vi "Main_Equip_Refo_ref749.vi"() -> ()   [LabVIEW 2017]
panel:
  out "TempeSenseTara":sgl caption="Temperature" format="%.1f"
  out "Temps SenseTara":sgl caption="Time" format="%.1f"
  out "TaraTemp":sgl[](array[numeric])
  in  "Test Selection":enum32{"Delta T", "EPI Calibration"}(radio)
  out "Pendent":sgl caption="Gradient :" format="%.2f"
  out "hardware name":string
  out "isOnline 2":bool
  out "IndexSup":i32
  out "IndexInf":i32
  in  "Verifica":bool
  out "High Time":sgl format="%#_3g"
  out "Low Time":sgl format="%#_3g"
  in  "High Temp.":sgl
  in  "Low Temp.":sgl
  out "Temps":sgl caption="Time" format="%.1f"
  out "Calibration result:":bool
  out "error out_USB":errorcluster
  out "Nom Sensor Temperatura":string
  in  "Dades":sgl[](array[numeric])
  in  "Guardar 24h":bool caption="Informe"
  out "Dies":u8 caption="NumDies"
  in  "Reset_AutoSave 24":bool
  in  "mT1":sgl caption="Temperatura_1" format="%.1f"
  out "Maxim":sgl
  in  "BtSalir":bool caption="Sortir"
  in  "Reset_AutoSave":bool
  in  "Test name:":string
  out "Gràfiques T-Temps":cluster{"Value":sgl[], "Value":sgl[]}[](graph)
  in  "Datos OK":bool
  out "DadesComplertes":sgl[](array[numeric])
  in  "Grafica_OK":bool=TRUE
  out "Tabla":sgl[][](array[numeric])
  in  "Registro OK":bool=TRUE
  in  "time out":bool
  in  "Reset_gráfica":bool
  in  "Reset_Time":bool
  in  "Tiempo_string":string[](array[string])
  out "Elapsed Time (s)":i32
  out "Ensayo activo":bool
  out "FSenseTara":sgl caption="Fuerza - N"
  in  "CaptadorF":u16(ring) caption="Unidades" items=["25kg"=5]
  in  "PendentLlum":sgl caption="Força" format="%.1f"
  out "FactorsUnitatsPendents_F":dbl[](array[numeric])
  out "ConversioUnitatsF":dbl[](array[numeric])=[1.0, 9.8756, 2.2]
  out "ArraiUnitats":cluster{"String":string, "Value":u16}[](array[cluster])=[{"String"="kg", "Value"=0}, {"String"="N", "Value"=1}, {"String"="g", "Value"=2}, {"String"="daN", "Value"=3}, {"String"="cN", "Value"=4}, {"String"="KN", "Value"=5}, {"String"="lb", "Value"=6}]
  out "Tara":sgl caption="Força" format="%.1f"
  out "Temperatura1":sgl caption="Temperature" format="%.1f"
  out "PendentsT":sgl[](array[numeric])
  in  "Salir":bool caption="Sortir"
  in  "Ensayonuevo":bool caption="New Test"
  in  "Guardar":bool
  in  "Iniciar / Finalizar":bool=TRUE caption="Finalitzar prova"
  in  "UnidadesF":u16(ring) caption="Unidades" items=["kg", "N", "g"]
  out "FirstTime?":bool caption="TARA"
  # "s"
  # "ºC / s"
  # "ºC"
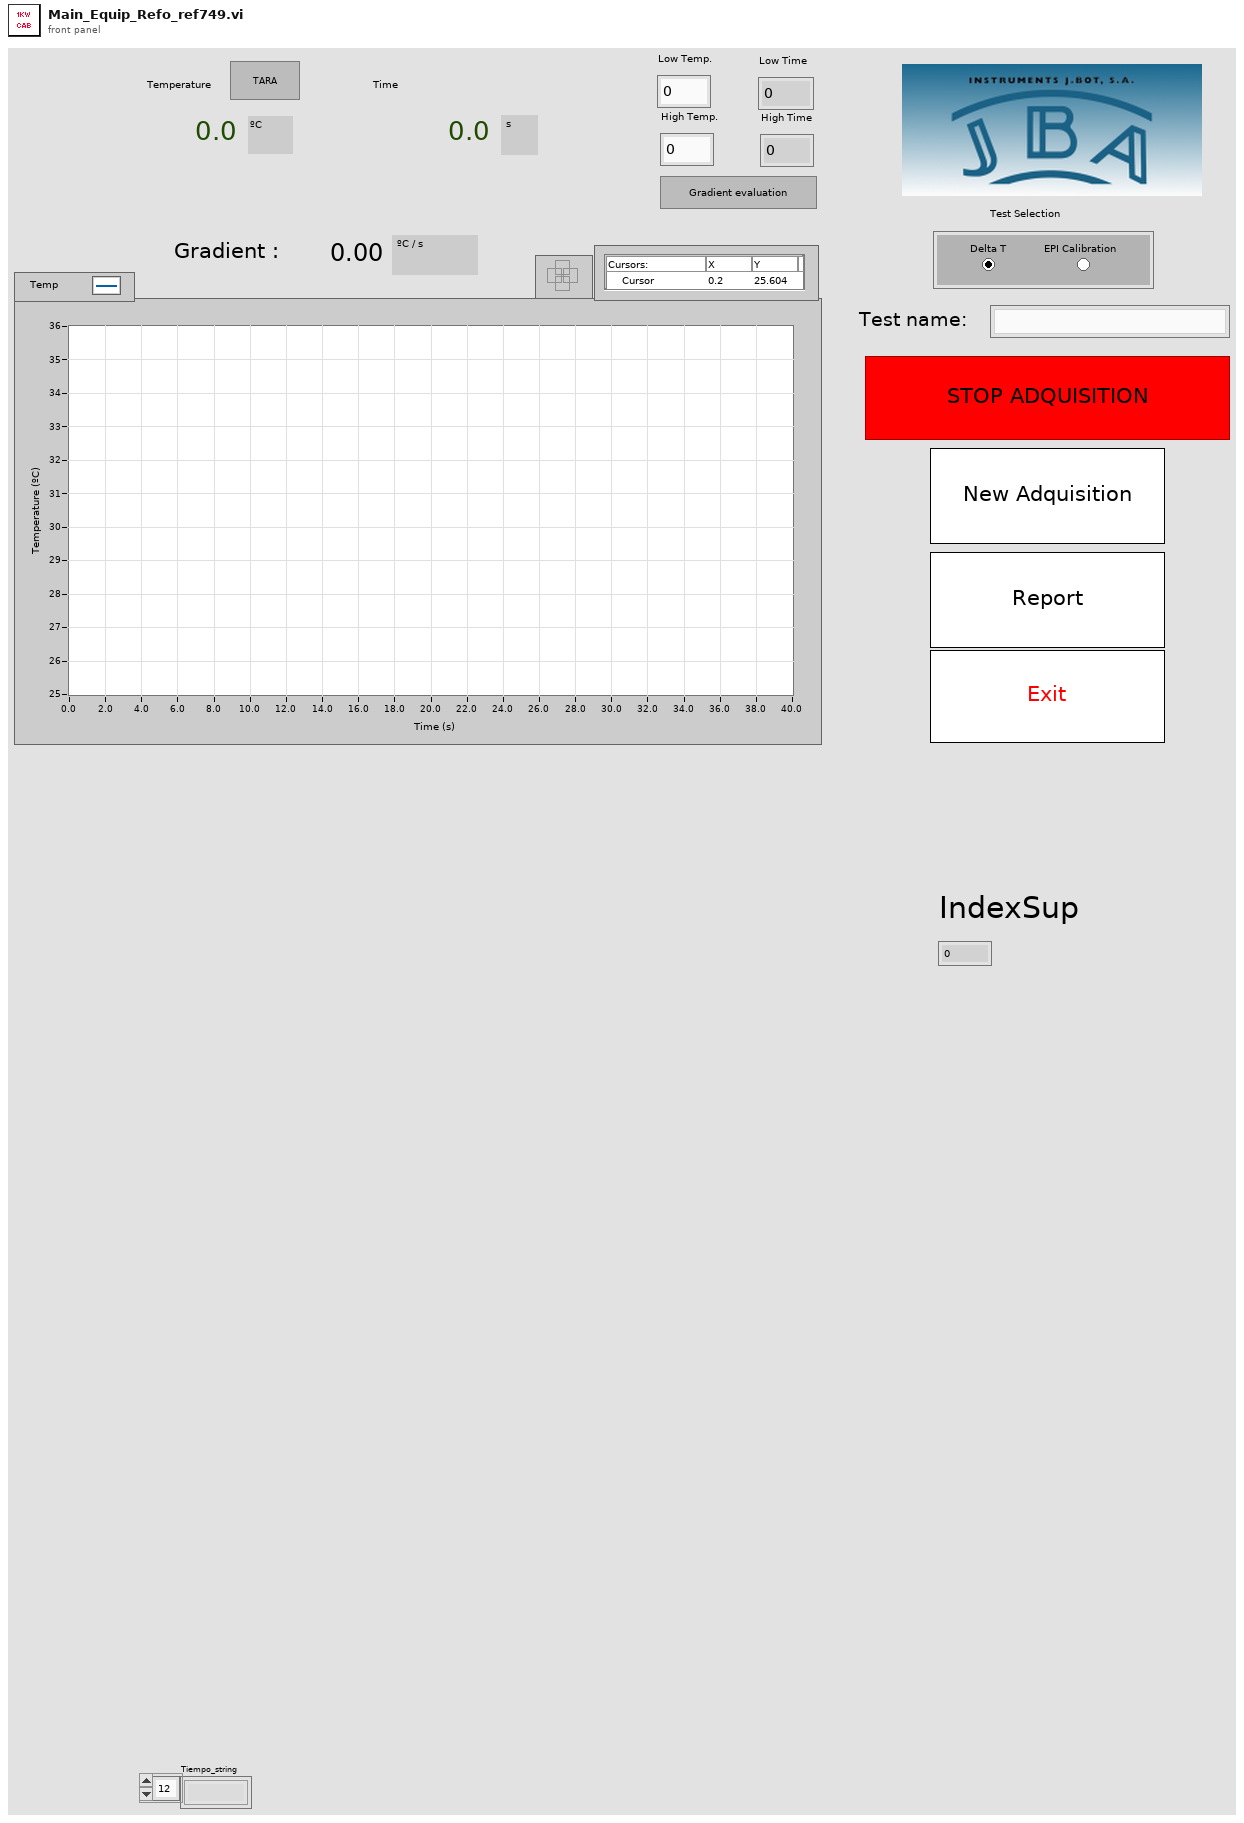
[diagram p1: front panel]
types:
  T1 = enum8{"Enabled", "Disabled", "Disabled and Grayed Out"}
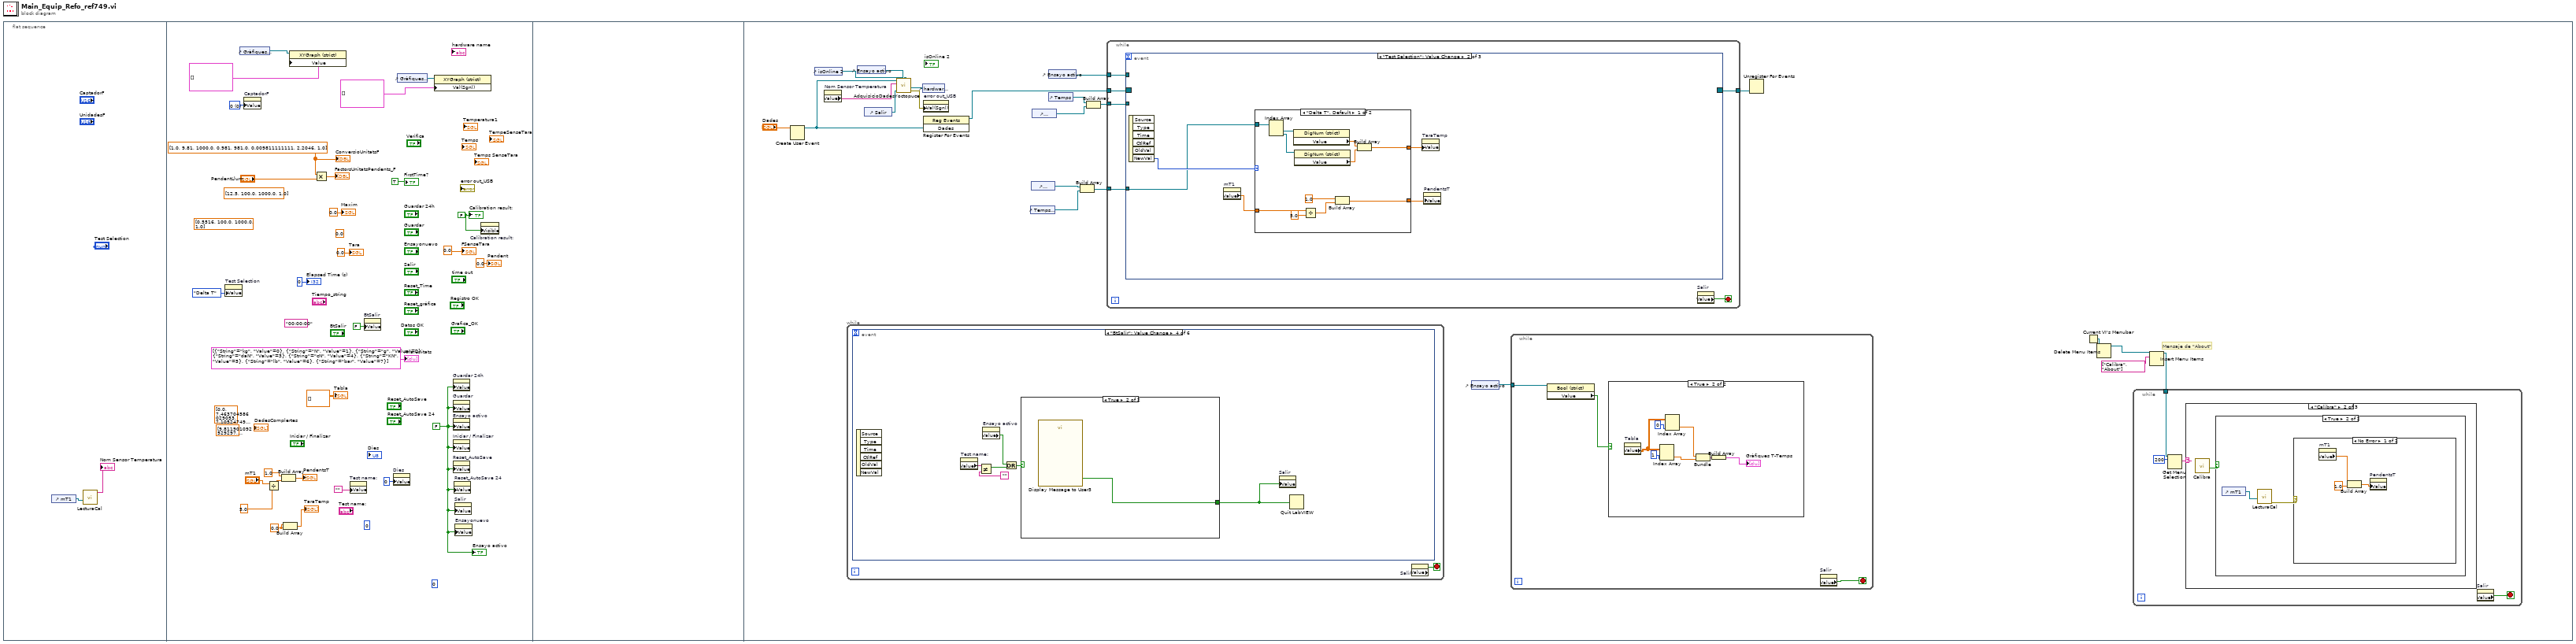
[diagram p0: block diagram]
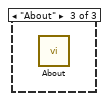
[diagram p5: hidden frame]
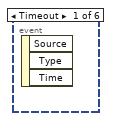
[diagram p7: hidden frame]
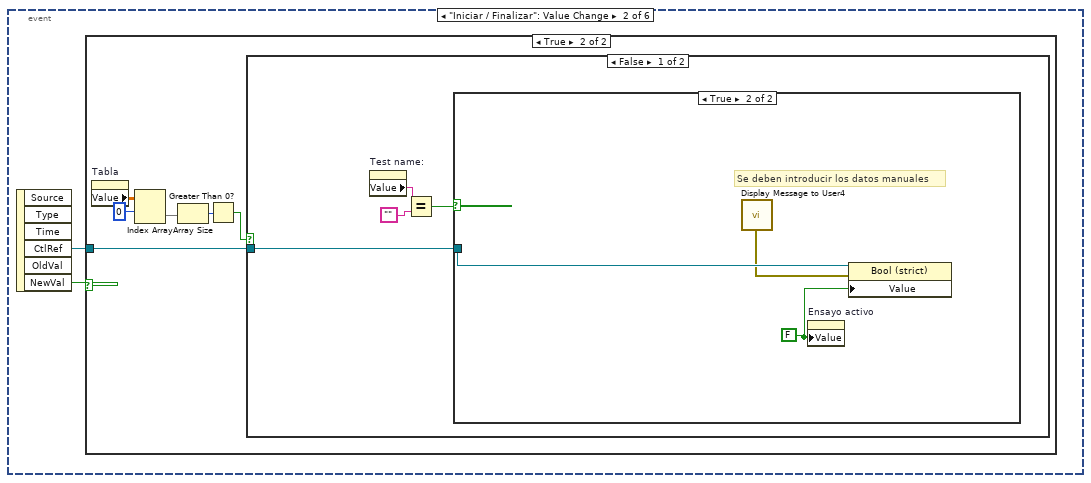
[diagram p8: hidden frame]
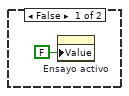
[diagram p9: hidden frame]
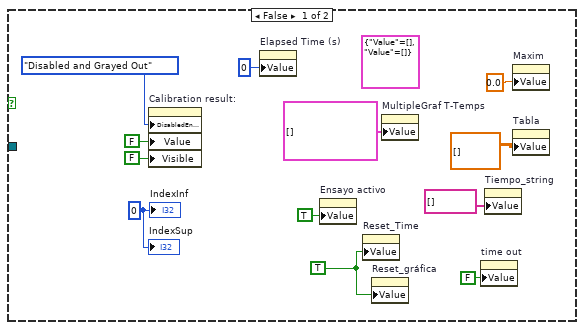
[diagram p10: hidden frame]
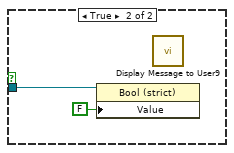
[diagram p11: hidden frame]
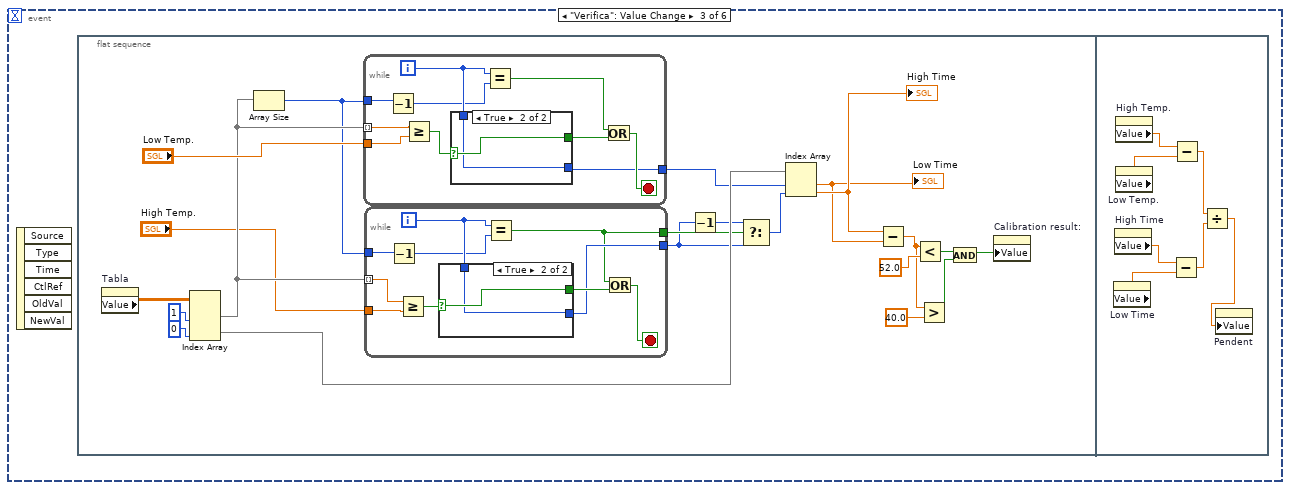
[diagram p12: hidden frame]
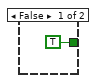
[diagram p15: hidden frame]
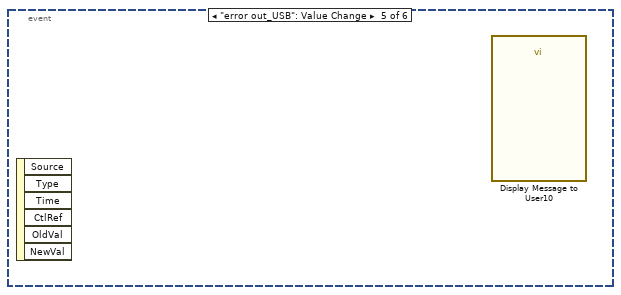
[diagram p16: hidden frame]
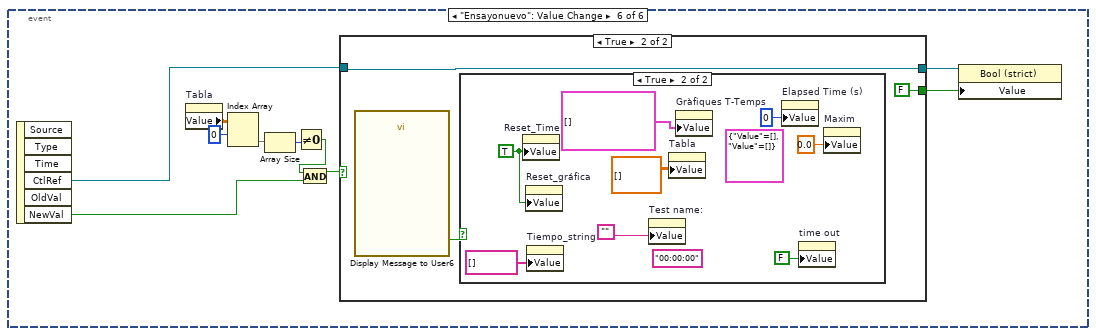
[diagram p17: hidden frame]
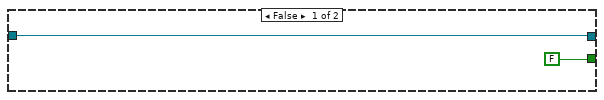
[diagram p18: hidden frame]
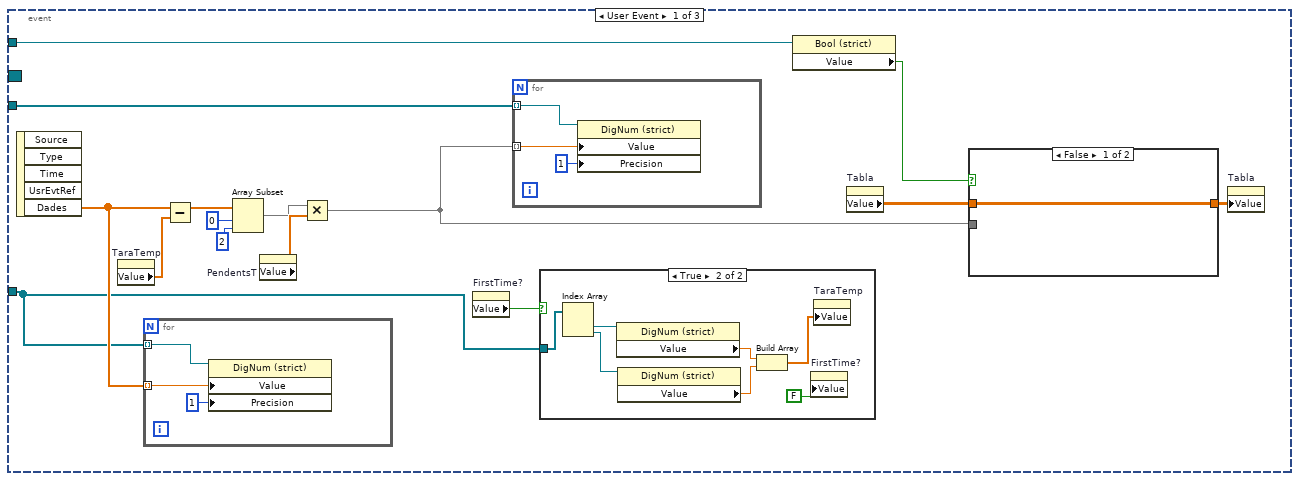
[diagram p20: hidden frame]
diagram:
  n1 = flat-sequence {
    frame #0 {
      n2 = control-ref of="mT1"() -> (w2:refnum<vi>)
      n3 = call "LecturaCal.vi"("T1"=w2) -> ("Nom Sensor Temperatura"=→"Nom Sensor Temperatura":string)  [unwired: 9 in, 1 out]
    }
    frame #1 {
      w10 = 0.0 ("element")
      w12 = FALSE ("Resultat Assaig")
      (unwired) sgl[] [9.811901, 9.763803, 9.671529, 9.535354] ("DadesComplertes")
      (unwired) sgl[][] [[0.0, 7.4637046, 7.1052475, 6.7309566, 6.297442], [5.0, 2.5386999, 2.902987, 3.276568, 3.6958933], [10.0, 7.471229, 7.101099, 6.7181377, 6.2959595], [15.0, 2.5153666, 2.9171765, 3.291629, 3.679636], [20.0, 7.4759755, 7.089289, 6.711311, 6.298526]] ("Tabla")
      (unwired) u8 0 ("Durada assaig minuts")
      (unwired) u8 0 ("Durada assaig - hores:")
      w22 = u16 0 items=["0"] ("CaptadorF")
      (unwired) sgl 0.0 ("Fuerza")
      (unwired) dbl[] [0.5516, 100.0, 1000.0, 1.0] ("y")
      (unwired) "00:00:00" ("Tiempo transcurrido (hh:mm:ss)")
      w13 = FALSE ("Ensayo activo")
      (unwired) dbl[] [12.5, 100.0, 1000.0, 1.0] ("y")
      w30 = dbl[] [1.0, 9.81, 1000.0, 0.981, 981.0, 0.009811111111, 2.2046, 1.0]
      n4 = property on="Test Selection" class="RadioBtnsControl (strict)"("Value"=enum32{"Delta T", "EPI Calibration"}."Delta T" ("Test Selection")) -> ()  [unwired: 2 in, 2 out]
      n5 = control-ref of="Gràfiques T-Temps"() -> (w15:refnum<vi>)
      n6 = property on="CaptadorF" class="Ring (strict)"("Value"=w22) -> ()  [unwired: 2 in, 2 out]
      n7 = Divide(x="mT1", y=sgl 5.0) -> (x/y=w4:sgl)
      n8 = Build Array(sgl 1.0 ("element"), w4) -> (→"PendentsT":sgl[])
      n9 = Build Array(w10, w10) -> (→"TaraTemp":dbl[])
      n10 = property class="XYGraph (strict)"(reference=w15, "Value"=cluster{"Value":sgl[], "Value":sgl[]}[] []) -> ()  [unwired: 1 in, 2 out]
      n11 = Multiply(x=w30, y="PendentLlum") -> (x*y=→"FactorsUnitatsPendents_F":dbl[])
      n12 = property on="Test name:" class="Str"("Value"="") -> ()  [unwired: 2 in, 2 out]
      n13 = property on="BtSalir" class="Bool (strict)"("Value"=FALSE ("BtSalir")) -> ()  [unwired: 2 in, 2 out]
      n14 = property on="Dies" class="DigNum (strict)"("Value"=u8 0 ("NumDies")) -> ()  [unwired: 2 in, 2 out]
      n15 = control-ref of="Gràfiques T-Temps"() -> (w18:refnum<vi>)
      n16 = property class="XYGraph (strict)"(reference=w18, "Val(Sgnl)"=cluster{"Value":sgl[], "Value":sgl[]}[] [] ("Value")) -> ()  [unwired: 1 in, 2 out]
      n17 = property on="Guardar 24h" class="Bool (strict)"("Value"=w13) -> ()  [unwired: 2 in, 2 out]
      n18 = property on="Guardar" class="Bool (strict)"("Value"=w13) -> ()  [unwired: 2 in, 2 out]
      n19 = property on="Ensayo activo" class="Bool (strict)"("Value"=w13) -> ()  [unwired: 2 in, 2 out]
      n20 = property on="Iniciar / Finalizar" class="Bool (strict)"("Value"=w13) -> ()  [unwired: 2 in, 2 out]
      n21 = property on="Reset_AutoSave" class="Bool (strict)"("Value"=w13) -> ()  [unwired: 2 in, 2 out]
      n22 = property on="Reset_AutoSave 24" class="Bool (strict)"("Value"=w13) -> ()  [unwired: 2 in, 2 out]
      n23 = property on="Salir" class="Bool (strict)"("Value"=w13) -> ()  [unwired: 2 in, 2 out]
      n24 = property on="Ensayonuevo" class="Bool (strict)"("Value"=w13) -> ()  [unwired: 2 in, 2 out]
      n25 = property on="Calibration result:" class="Bool (strict)"("Visible"=w12) -> ()  [unwired: 2 in, 2 out]
      "FirstTime?" <- TRUE ("FirstTime?")
      "Tara" <- sgl 0.0 ("Tara")
      "ArraiUnitats" <- cluster{"String":string, "Value":u16}[] [{"String"="kg", "Value"=0}, {"String"="N", "Value"=1}, {"String"="g", "Value"=2}, {"String"="daN", "Value"=3}, {"String"="cN", "Value"=4}, {"String"="KN", "Value"=5}, {"String"="lb", "Value"=6}, {"String"="bar", "Value"=7}] ("Strings And Values [] 2")
      "ConversioUnitatsF" <- w30
      "FSenseTara" <- sgl 0.0 ("FSenseTara")
      "Elapsed Time (s)" <- 0 ("Elapsed Time (s)")
      "Tabla" <- sgl[][] [] ("Tabla")
      "Maxim" <- sgl 0.0 ("Maxim")
      "Calibration result:" <- w12
      "Ensayo activo" <- w13
      "Pendent" <- sgl 0.0 ("Pendent")
    }
    frame #2 {
    }
    frame #3 {
      # "Mensaje de \"About\""
      n26 = Create User Event(user event datatype="Dades") -> (user event=w42:refnum<user-event>)  [unwired: 1 in, 1 out]
      n27 = control-ref of="isOnline 2"() -> (w38:refnum<vi>)
      n28 = property on="Nom Sensor Temperatura" class="Str"() -> ("Value"=w41:string)  [unwired: 2 in, 2 out]
      n29 = while {
        stop <- w74 stop-if-true
        n30 = event shown="[3] \"BtSalir\": Value Change" {
          selector: _ -> [_ _ _ _ _ _]
          dyn-events: _ -> [_ _ _ _ _ _]
          timeout: _ -> [_ _ _ _ _ _]
          event Timeout {
            n31 = event-data() -> ()  [unwired: 1 in, 3 out]
          }
          event "Iniciar / Finalizar": Value Change {
            n32 = event-data() -> ("CtlRef"=w75:refnum<vi>, "NewVal"=w76:bool)  [unwired: 1 in, 4 out]
            n33 = case shown="True" w76 {
              tunnel: w75 -> [_ w83]
              frame False {
                n34 = property on="Ensayo activo" class="Bool (strict)"("Value"=FALSE ("Ensayo activo")) -> ()  [unwired: 2 in, 2 out]
              }
              frame True {
                n35 = property on="Tabla" class="Arr (strict)"() -> ("Value"=w82:sgl[][])  [unwired: 2 in, 2 out]
                n36 = Index Array(array=w82, index (row)=0) -> (element=w81:sgl[])  [unwired: 1 in]
                n37 = Array Size(array=w81) -> (size(s)=w79:i32)
                n38 = Greater Than 0?(x=w79) -> (x > 0?=w78:bool)
                n39 = case shown="False" w78 {
                  tunnel: w83 -> [w87 w104]
                  frame False {
                    n40 = property on="Test name:" class="Str"() -> ("Value"=w86:string)  [unwired: 2 in, 2 out]
                    n41 = Equal?(x=w86, y="") -> (x = y?=w84:bool)
                    n42 = case shown="True" w84 {
                      tunnel: w87 -> [_ w102]
                      frame False {
                        w88 = 0 ("IndexInf")
                        (unwired) cluster{"Value":sgl[], "Value":sgl[]} {"Value"=[], "Value"=[]} ("Grafica F-T")
                        w97 = TRUE ("Reset_Time")
                        n43 = property on="Calibration result:" class="Bool (strict)"("DisabledEnum"=T1."Disabled and Grayed Out" ("Disabled"), "Value"=FALSE ("Resultat Assaig"), "Visible"=FALSE) -> ()  [unwired: 2 in, 2 out]
                        n44 = property on="Elapsed Time (s)" class="DigNum (strict)"("Value"=0 ("Elapsed Time (s)")) -> ()  [unwired: 2 in, 2 out]
                        n45 = property on="Ensayo activo" class="Bool (strict)"("Value"=TRUE ("Iniciar assaig")) -> ()  [unwired: 2 in, 2 out]
                        n46 = property on="Reset_Time" class="Bool (strict)"("Value"=w97) -> ()  [unwired: 2 in, 2 out]
                        n47 = property on="Reset_gráfica" class="Bool (strict)"("Value"=w97) -> ()  [unwired: 2 in, 2 out]
                        n48 = property on="MultipleGraf T-Temps" class="XYGraph (strict)"("Value"=cluster{"Y":dbl[], "Y":dbl[]}[] []) -> ()  [unwired: 2 in, 2 out]
                        n49 = property on="time out" class="Bool (strict)"("Value"=FALSE ("time out")) -> ()  [unwired: 2 in, 2 out]
                        n50 = property on="Tiempo_string" class="Arr (strict)"("Value"=string[] [] ("Tiempo_string")) -> ()  [unwired: 2 in, 2 out]
                        n51 = property on="Maxim" class="DigNum (strict)"("Value"=sgl 0.0 ("Maxim")) -> ()  [unwired: 2 in, 2 out]
                        n52 = property on="Tabla" class="Arr (strict)"("Value"=sgl[][] [] ("Tabla")) -> ()  [unwired: 2 in, 2 out]
                        "IndexSup" <- w88
                        "IndexInf" <- w88
                      }
                      frame True {
                        w101 = FALSE
                        # "Se deben introducir los datos manuales"
                        n53 = call "Display Message to User4"() -> ("error out"=w100:errorcluster)  [unwired: 10 in, 1 out]
                        n54 = property on="Ensayo activo" class="Bool (strict)"("Value"=w101) -> ()  [unwired: 2 in, 2 out]
                        n55 = property class="Bool (strict)"(reference=w102, error in=w100, "Value"=w101) -> ()  [unwired: 2 out]
                      }
                    }
                  }
                  frame True {
                    n56 = property class="Bool (strict)"(reference=w104, "Value"=FALSE) -> ()  [unwired: 1 in, 2 out]
                    n57 = call "Display Message to User9"() -> ()  [unwired: 10 in, 2 out]
                  }
                }
              }
            }
          }
          event "Verifica": Value Change {
            n58 = event-data() -> ()  [unwired: 1 in, 6 out]
            n59 = flat-sequence {
              frame #0 {
                n60 = property on="Tabla" class="Arr (strict)"() -> ("Value"=w125:sgl[][])  [unwired: 2 in, 2 out]
                n61 = Index Array(array=w125, index (col) #1=1 ("index (row)"), index (col) #2=0 ("index (row)")) -> (element #1=w118:sgl[], element #2=w115:sgl[])  [unwired: 2 in]
                n62 = Array Size(array=w118) -> (size(s)=w116:i32)
                n63 = while {
                  tunnel: w118 -> [w148] mode=indexing
                  tunnel: "Low Temp." -> [w147]
                  tunnel: w116 -> [w144]
                  tunnel: [w139] -> w114
                  i -> [w145]
                  stop <- w140 stop-if-true
                  n64 = Decrement(x=w144) -> (x-1=w143:i32)
                  n65 = Greater Or Equal?(x=w148, y=w147) -> (x >= y?=w146:bool)
                  n66 = case shown="True" w146 {
                    selector: w146 -> [w149 w151]
                    tunnel: w145 -> [_ w150]
                    tunnel: [w149 w151] -> w141
                    tunnel: [_ w150] -> w139
                    frame False {
                    }
                    frame True {
                    }
                  }
                  n67 = Equal?(x=w145, y=w143) -> (x = y?=w142:bool)
                  n68 = Or(x=w142, y=w141) -> (x .or. y?=w140:bool)
                }
                n69 = while {
                  tunnel: w118 -> [w135] mode=indexing
                  tunnel: "High Temp." -> [w129]
                  tunnel: w116 -> [w128]
                  tunnel: [w127] -> w105
                  tunnel: [w126] -> w108
                  i -> [w133]
                  stop <- w130 stop-if-true
                  n70 = Decrement(x=w128) -> (x-1=w132:i32)
                  n71 = Greater Or Equal?(x=w135, y=w129) -> (x >= y?=w134:bool)
                  n72 = case shown="True" w134 {
                    selector: w134 -> [w136 w138]
                    tunnel: w133 -> [_ w137]
                    tunnel: [w136 w138] -> w131
                    tunnel: [_ w137] -> w127
                    frame False {
                    }
                    frame True {
                    }
                  }
                  n73 = Equal?(x=w133, y=w132) -> (x = y?=w126:bool)
                  n74 = Or(x=w126, y=w131) -> (x .or. y?=w130:bool)
                }
                n75 = Decrement(x=w105) -> (x-1=w106:i32)
                n76 = Select(t=w106, s=w108, f=w105) -> (s? t:f=w107:i32)
                n77 = Index Array(array=w115, index #1=w114, index #2=w107) -> (element #1=w122:sgl, element #2=w123:sgl)
                "Low Time" <- w122
                "High Time" <- w123
                n78 = Subtract(x=w123, y=w122) -> (x-y=w112:sgl)
                n79 = Less?(x=w112, y=sgl 52.0) -> (x < y?=w110:bool)
                n80 = Greater?(x=w112, y=40.0) -> (0:w109:bool)
                n81 = And(x=w110, y=w109) -> (x .and. y?=w111:bool)
                n82 = property on="Calibration result:" class="Bool (strict)"("Value"=w111) -> ()  [unwired: 2 in, 2 out]
              }
              frame #1 {
                n83 = property on="Low Time" class="DigNum (strict)"() -> ("Value"=w155:sgl)  [unwired: 2 in, 2 out]
                n84 = property on="High Time" class="DigNum (strict)"() -> ("Value"=w156:sgl)  [unwired: 2 in, 2 out]
                n85 = property on="High Temp." class="DigNum (strict)"() -> ("Value"=w158:sgl)  [unwired: 2 in, 2 out]
                n86 = property on="Low Temp." class="DigNum (strict)"() -> ("Value"=w157:sgl)  [unwired: 2 in, 2 out]
                n87 = Subtract(x=w156, y=w155) -> (x-y=w153:sgl)
                n88 = Subtract(x=w158, y=w157) -> (x-y=w154:sgl)
                n89 = Divide(x=w154, y=w153) -> (x/y=w152:sgl)
                n90 = property on="Pendent" class="DigNum (strict)"("Value"=w152) -> ()  [unwired: 2 in, 2 out]
              }
            }
          }
          event "BtSalir": Value Change {
            n91 = event-data() -> ()  [unwired: 1 in, 6 out]
            n92 = property on="Test name:" class="Str"() -> ("Value"=w163:string)  [unwired: 2 in, 2 out]
            n93 = Not Equal?(x=w163, y="") -> (x != y?=w159:bool)
            n94 = property on="Ensayo activo" class="Bool (strict)"() -> ("Value"=w160:bool)  [unwired: 2 in, 2 out]
            n95 = Or(x=w160, y=w159) -> (x .or. y?=w161:bool)
            n96 = case shown="True" w161 {
              tunnel: [TRUE ("OK") w166] -> w164
              frame False {
              }
              frame True {
                n97 = call "Display Message to User3"() -> ("OK"=w166:bool)  [unwired: 10 in, 1 out]
              }
            }
            n98 = property on="Salir" class="Bool (strict)"("Value"=w164) -> ()  [unwired: 2 in, 2 out]
            n99 = Quit LabVIEW(quit? (T)=w164) -> ()
          }
          event "error out_USB": Value Change {
            n100 = event-data() -> ()  [unwired: 1 in, 6 out]
            n101 = call "Display Message to User10"() -> ()  [unwired: 10 in, 2 out]
          }
          event "Ensayonuevo": Value Change {
            n102 = event-data() -> ("CtlRef"=w174:refnum<vi>, "NewVal"=w167:bool)  [unwired: 1 in, 4 out]
            n103 = property on="Tabla" class="Arr (strict)"() -> ("Value"=w172:sgl[][])  [unwired: 2 in, 2 out]
            n104 = Index Array(array=w172, index (row)=0) -> (element=w169:sgl[])  [unwired: 1 in]
            n105 = Array Size(array=w169) -> (size(s)=w170:i32)
            n106 = Not Equal To 0?(x=w170) -> (x != 0?=w168:bool)
            n107 = And(x=w168, y=w167) -> (x .and. y?=w173:bool)
            n108 = case shown="True" w173 {
              tunnel: w174 -> [w178 w180]
              tunnel: [w178 w180] -> w175
              tunnel: [FALSE ("Value") FALSE ("Value")] -> w176
              frame False {
              }
              frame True {
                n109 = call "Display Message to User6"() -> ("Yes"=w181:bool)  [unwired: 10 in, 1 out]
                n110 = case shown="True" w181 {
                  frame False {
                  }
                  frame True {
                    (unwired) "00:00:00" ("Tiempo transcurrido (hh:mm:ss)")
                    w186 = TRUE ("Reset_Time")
                    (unwired) cluster{"Value":sgl[], "Value":sgl[]} {"Value"=[], "Value"=[]} ("Grafica F-T")
                    n111 = property on="Reset_Time" class="Bool (strict)"("Value"=w186) -> ()  [unwired: 2 in, 2 out]
                    n112 = property on="Reset_gráfica" class="Bool (strict)"("Value"=w186) -> ()  [unwired: 2 in, 2 out]
                    n113 = property on="Tiempo_string" class="Arr (strict)"("Value"=string[] [] ("Tiempo_string")) -> ()  [unwired: 2 in, 2 out]
                    n114 = property on="Test name:" class="Str"("Value"="") -> ()  [unwired: 2 in, 2 out]
                    n115 = property on="Tabla" class="Arr (strict)"("Value"=sgl[][] [] ("Tabla")) -> ()  [unwired: 2 in, 2 out]
                    n116 = property on="Gràfiques T-Temps" class="XYGraph (strict)"("Value"=cluster{"Y":dbl[], "Y":dbl[]}[] []) -> ()  [unwired: 2 in, 2 out]
                    n117 = property on="Elapsed Time (s)" class="DigNum (strict)"("Value"=0 ("Elapsed Time (s)")) -> ()  [unwired: 2 in, 2 out]
                    n118 = property on="time out" class="Bool (strict)"("Value"=FALSE ("time out")) -> ()  [unwired: 2 in, 2 out]
                    n119 = property on="Maxim" class="DigNum (strict)"("Value"=sgl 0.0 ("Maxim")) -> ()  [unwired: 2 in, 2 out]
                  }
                }
              }
            }
            n120 = property class="Bool (strict)"(reference=w175, "Value"=w176) -> ()  [unwired: 1 in, 2 out]
          }
        }
        n121 = property on="Salir" class="Bool (strict)"() -> ("Value"=w74:bool)  [unwired: 2 in, 2 out]
      }
      n122 = control-ref of="Ensayo activo"() -> (w39:refnum<vi>)
      n123 = control-ref of="Salir"() -> (w43:refnum<vi>)
      n124 = control-ref of="hardware name"() -> (w37:refnum<vi>)
      n125 = call "AdquisicioDadesYoctopuce.vi"("HardName"=w37, "online?"=w38, "AssaigActiu"=w39, "Stop"=w43, "Temperature name"=w41, "user event in"=w42) -> ("error out"=w40:errorcluster)  [unwired: 4 in, 1 out]
      n126 = property on="error out_USB" class="Clust (strict)"("Val(Sgnl)"=w40) -> ()  [unwired: 2 in, 2 out]
      n127 = register-events(w42) -> (reference out=w35:refnum<event-registration>)  [unwired: 2 in, 1 out]
      n128 = control-ref of="Temps SenseTara"() -> (w33:refnum<vi>)
      n129 = control-ref of="TempeSenseTara"() -> (w34:refnum<vi>)
      n130 = control-ref of="Temperatura1"() -> (w44:refnum<vi>)
      n131 = control-ref of="Ensayo activo"() -> (w47:refnum<vi>)
      n132 = control-ref of="Temps"() -> (w45:refnum<vi>)
      n133 = Build Array(w34, w33) -> (w32:refnum<vi>[])
      n134 = Build Array(w45, w44) -> (w48:refnum<vi>[])
      n135 = while {
        tunnel: [w195] -> w53
        tunnel: w48 -> [w193]
        tunnel: w47 -> [w192]
        tunnel: w35 -> [w191]
        tunnel: w32 -> [w190]
        stop <- w194 stop-if-true
        n136 = event shown="[1] \"Test Selection\": Value Change" {
          selector: w191 -> [_ _ _]
          dyn-events: [_ _ _] -> w195
          timeout: _ -> [_ _ _]
          tunnel: w193 -> [w197 _ _]
          tunnel: w192 -> [w207 _ _]
          tunnel: w190 -> [w196 w228 _]
          event User Event {
            n137 = event-data() -> ("Dades"=w201:sgl[])  [unwired: 1 in, 4 out]
            n138 = property on="TaraTemp" class="Arr (strict)"() -> ("Value"=w198:sgl[])  [unwired: 2 in, 2 out]
            n139 = for {
              tunnel: w196 -> [w211] mode=indexing
              tunnel: w201 -> [w212] mode=indexing
              n140 = property class="DigNum (strict)"(reference=w211, "Value"=w212, "Precision"=u8 1 ("Display Format:Precision")) -> ()  [unwired: 1 in, 2 out]
            }
            n141 = Subtract(x=w201, y=w198) -> (x-y=w199:sgl[])
            n142 = Array Subset(array=w199, index=0, length=2) -> (w203:sgl[])
            n143 = property on="PendentsT" class="Arr (strict)"() -> ("Value"=w208:sgl[])  [unwired: 2 in, 2 out]
            n144 = Multiply(x=w203, y=w208) -> (x*y=w200:sgl[])
            n145 = property on="FirstTime?" class="Bool (strict)"() -> ("Value"=w202:bool)  [unwired: 2 in, 2 out]
            n146 = for {
              tunnel: w197 -> [w221] mode=indexing
              tunnel: w200 -> [w222] mode=indexing
              n147 = property class="DigNum (strict)"(reference=w221, "Value"=w222, "Precision"=u8 1 ("Display Format:Precision")) -> ()  [unwired: 1 in, 2 out]
            }
            n148 = case shown="True" w202 {
              tunnel: w196 -> [_ w215]
              frame False {
              }
              frame True {
                n149 = Index Array(array=w215) -> (element #1=w219:refnum<vi>, element #2=w218:refnum<vi>)  [unwired: 2 in]
                n150 = property class="DigNum (strict)"(reference=w219) -> ("Value"=w217:sgl)  [unwired: 1 in, 2 out]
                n151 = property class="DigNum (strict)"(reference=w218) -> ("Value"=w216:sgl)  [unwired: 1 in, 2 out]
                n152 = Build Array(w217, w216) -> (w214:sgl[])
                n153 = property on="FirstTime?" class="Bool (strict)"("Value"=FALSE ("FirstTime?")) -> ()  [unwired: 2 in, 2 out]
                n154 = property on="TaraTemp" class="Arr (strict)"("Value"=w214) -> ()  [unwired: 2 in, 2 out]
              }
            }
            n155 = property class="Bool (strict)"(reference=w207) -> ("Value"=w206:bool)  [unwired: 1 in, 2 out]
            n156 = property on="Tabla" class="Arr (strict)"() -> ("Value"=w205:sgl[][])  [unwired: 2 in, 2 out]
            n157 = case shown="False" w206 {
              tunnel: w200 -> [_ w227]
              tunnel: w205 -> [w224 w226]
              tunnel: [w224 w225] -> w204
              frame False {
              }
              frame True {
                n158 = Build Array (concatenate)(w226, w227) -> (w225:sgl[][])
              }
            }
            n159 = property on="Tabla" class="Arr (strict)"("Value"=w204) -> ()  [unwired: 2 in, 2 out]
          }
          event "Test Selection": Value Change {
            n160 = event-data() -> ("NewVal"=w232:enum32{"Delta T", "EPI Calibration"})  [unwired: 1 in, 5 out]
            n161 = property on="mT1" class="DigNum (strict)"() -> ("Value"=w229:sgl)  [unwired: 2 in, 2 out]
            n162 = case shown="\"Delta T\", Default" w232 {
              tunnel: w228 -> [w243 _]
              tunnel: [w238 w247] -> w231
              tunnel: [w233 w244] -> w230
              tunnel: w229 -> [w236 w245]
              frame "Delta T", Default {
                n163 = Index Array(array=w243) -> (element #1=w242:refnum<vi>, element #2=w241:refnum<vi>)  [unwired: 2 in]
                n164 = property class="DigNum (strict)"(reference=w242) -> ("Value"=w240:sgl)  [unwired: 1 in, 2 out]
                n165 = property class="DigNum (strict)"(reference=w241) -> ("Value"=w239:sgl)  [unwired: 1 in, 2 out]
                n166 = Divide(x=w236, y=sgl 5.0) -> (x/y=w234:sgl)
                n167 = Build Array(1.0 ("element"), w234) -> (w233:dbl[])
                n168 = Build Array(w240, w239) -> (w238:sgl[])
              }
              frame "EPI Calibration" {
                w248 = 0.0 ("element")
                n169 = Build Array(w248, w248) -> (w247:dbl[])
                n170 = Build Array(1.0 ("element"), w245) -> (w244:dbl[])
              }
            }
            n171 = property on="TaraTemp" class="Arr (strict)"("Value"=w231) -> ()  [unwired: 2 in, 2 out]
            n172 = property on="PendentsT" class="Arr (strict)"("Value"=w230) -> ()  [unwired: 2 in, 2 out]
          }
          event "Guardar": Value Change {
            n173 = event-data() -> ("CtlRef"=w249:refnum<vi>, "NewVal"=w251:bool)  [unwired: 1 in, 4 out]
            n174 = case shown="True" w251 {
              tunnel: [errorcluster {"status"=FALSE, "code"=0, "source"=""} ("error out") w271] -> w250
              tunnel: w249 -> [_ w261]
              frame False {
              }
              frame True {
                n175 = property on="Tabla" class="Arr (strict)"() -> ("Value"=w255:sgl[][])  [unwired: 2 in, 2 out]
                n176 = Index Array(array=w255, index (row)=0) -> (element=w269:sgl[])  [unwired: 1 in]
                n177 = property class="Bool (strict)"(reference=w261, "BoolText.Text"="Generating report" ("Boolean Text.Text")) -> (reference out=w260:refnum<vi>, error out=w256:errorcluster)  [unwired: 1 in]
                n178 = Array Size(array=w269) -> (size(s)=w257:i32)
                n179 = Not Equal To 0?(x=w257) -> (x != 0?=w268:bool)
                n180 = flat-sequence {
                  tunnel: w255 -> [w277]
                  tunnel: w268 -> [w276]
                  tunnel: w260 -> [w274]
                  tunnel: [w278] -> w264
                  tunnel: [w275] -> w263
                  tunnel: [w273] -> w262
                  tunnel: w256 -> [w272]
                  tunnel: [w289] -> w266
                  tunnel: [w290] -> w267
                  tunnel: [w291] -> w271
                  tunnel: w264 -> [w291]
                  tunnel: w263 -> [w290]
                  tunnel: w262 -> [w289]
                  frame #0 {
                    n181 = case shown="True" w276 {
                      tunnel: [errorcluster {"status"=TRUE, "code"=0, "source"=""} ("error out") w284] -> w278
                      tunnel: w277 -> [_ w286]
                      tunnel: [w280 w283] -> w275
                      tunnel: w274 -> [w279 w287]
                      tunnel: [w279 w287] -> w273
                      tunnel: w272 -> [_ w283]
                      frame False {
                        n182 = call "Display Message to User8"() -> ("error out"=w280:errorcluster)  [unwired: 10 in, 1 out]
                      }
                      frame True {
                        n183 = property on="Test name:" class="Str"() -> ("Value"=w285:string)  [unwired: 2 in, 2 out]
                        n184 = call "CreaInformeExcel.vi"("Nom Assaig"=w285, "NºTests"=u8 1, "Tabla"=w286) -> ("error out"=w284:errorcluster)  [unwired: 15 in, 1 out]
                      }
                    }
                  }
                  frame #1 {
                    n185 = Wait Until Next ms Multiple(millisecond multiple=u32 200 ("milliseconds to wait")) -> ()  [unwired: 1 out]
                  }
                }
                n186 = property class="Bool (strict)"(reference=w266, error in=w267, "Value"=FALSE, "BoolText.Text"="Report" ("Boolean Text.Text")) -> ()  [unwired: 2 out]
              }
            }
            n187 = case shown="No Error" w250 {
              selector: w250 -> [w252 _]
              frame No Error {
                n188 = case shown="No Error" w252 {
                  frame No Error {
                    n189 = call "Display Message to User5"() -> ()  [unwired: 10 in, 2 out]
                  }
                  frame Error {
                    n190 = property on="Reset_AutoSave" class="Bool (strict)"("Value"=FALSE ("Reset_AutoSave")) -> ()  [unwired: 2 in, 2 out]
                  }
                }
              }
              frame Error {
              }
            }
          }
        }
        n191 = property on="Salir" class="Bool (strict)"() -> ("Value"=w194:bool)  [unwired: 2 in, 2 out]
      }
      n192 = control-ref of="Ensayo activo"() -> (w46:refnum<vi>)
      n193 = while {
        tunnel: w46 -> [w65]
        stop <- w66 stop-if-true
        n194 = property class="Bool (strict)"(reference=w65) -> ("Value"=w64:bool)  [unwired: 1 in, 2 out]
        n195 = case shown="True" w64 {
          frame False {
          }
          frame True {
            n196 = property on="Tabla" class="Arr (strict)"() -> ("Value"=w69:sgl[][])  [unwired: 2 in, 2 out]
            n197 = Index Array(array=w69, index (col)=1 ("index")) -> (element=w68:sgl[])  [unwired: 1 in]
            n198 = Index Array(array=w69, index (col)=0 ("index (row)")) -> (element=w67:sgl[])  [unwired: 1 in]
            n199 = Bundle("Value"=w67, "Value"=w68) -> (w73:cluster{"Value":sgl[], "Value":sgl[]})  [unwired: 1 in]
            n200 = Build Array(w73) -> (→"Gràfiques T-Temps":cluster{"Value":sgl[], "Value":sgl[]}[])
          }
        }
        n201 = property on="Salir" class="Bool (strict)"() -> ("Value"=w66:bool)  [unwired: 2 in, 2 out]
      }
      n202 = Unregister For Events(event registration refnum=w53) -> ()  [unwired: 1 in, 1 out]
      n203 = Current VI's Menubar() -> (w52:refnum<k9>)
      n204 = Delete Menu Items(9:w52) -> (3:w51:refnum<k9>)  [unwired: 3 in, 1 out]
      n205 = Insert Menu Items(8:string[] ["Calibra", "About"] ("item names"), 9:w51) -> (3:w50:refnum<k9>)  [unwired: 4 in, 2 out]
      n206 = while {
        tunnel: w50 -> [w55]
        stop <- w57 stop-if-true
        n207 = Get Menu Selection(0:w55, 1:200 ("ms timeout (200)")) -> (6:w54:string)  [unwired: 2 in, 4 out]
        n208 = case shown="\"Calibra\"" w54 {
          frame "False", Default {
          }
          frame "Calibra" {
            n209 = call "Calibra.vi"() -> ("SurtOk?"=w58:bool)  [unwired: 11 in]
            n210 = case shown="True" w58 {
              frame False {
              }
              frame True {
                n211 = control-ref of="mT1"() -> (w60:refnum<vi>)
                n212 = call "LecturaCal.vi"("T1"=w60) -> ("error out"=w59:errorcluster)  [unwired: 9 in, 1 out]
                n213 = case shown="No Error" w59 {
                  frame No Error {
                    n214 = property on="mT1" class="DigNum (strict)"() -> ("Value"=w63:sgl)  [unwired: 2 in, 2 out]
                    n215 = Build Array(w63, sgl 1.0 ("element")) -> (w62:sgl[])
                    n216 = property on="PendentsT" class="Arr (strict)"("Value"=w62) -> ()  [unwired: 2 in, 2 out]
                  }
                  frame Error {
                  }
                }
              }
            }
          }
          frame "About" {
            n217 = call "About.vi"() -> ()  [unwired: 1 in]
          }
        }
        n218 = property on="Salir" class="Bool (strict)"() -> ("Value"=w57:bool)  [unwired: 2 in, 2 out]
      }
    }
  }
